vi "Timer Off Delay（SM).vi"(8 "error in":errorcluster caption="error IO", 10 "preset time (ms)":u32=1000, 11 "input":bool) -> (0 "error out":errorcluster caption="error IO", 2 "elapsed time (ms)":u32, 3 "output":bool)   [LabVIEW 2012, in "毫秒定时器.lvlib"]
uses:
  <vilib>/ptbypt/NI_PtbyPt.lvlib
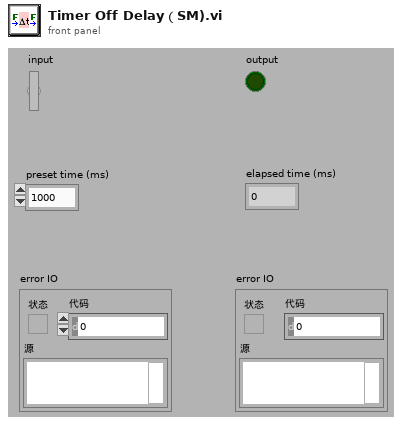
[diagram p1: front panel]
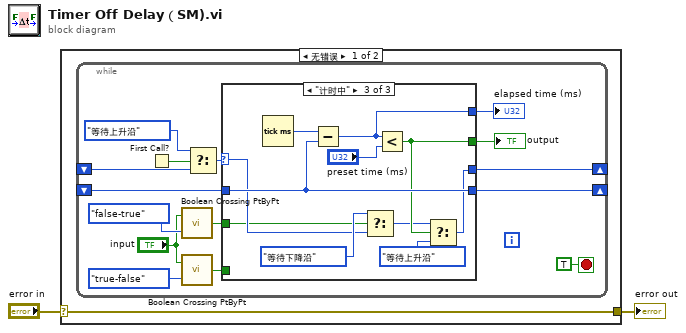
[diagram p0: block diagram]
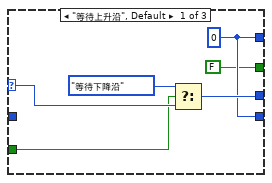
[diagram p2: hidden frame]
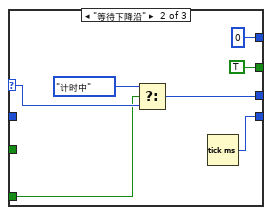
[diagram p3: hidden frame]
diagram:
  n1 = case shown="无错误" "error in" {
    selector: "error in" -> [w3 w43]
    tunnel: [w3 w43] -> w2
    frame No Error {
      n2 = while {
        shift-right: [w10] -> _
        shift-left: _ -> [w17]
        shift-right: [w11] -> _
        shift-left: _ -> [w13]
        stop <- TRUE stop-if-true
        n3 = First Call?() -> (First Call?: T/F=w16:bool)
        n4 = call <vilib>:"Boolean Crossing PtByPt.vi"("direction"=enum16{"either", "false-true", "true-false"}."false-true", "input"="input") -> ("crossing"=w5:bool)  [unwired: 1 in]
        n5 = call <vilib>:"Boolean Crossing PtByPt.vi"("direction"=enum16{"either", "false-true", "true-false"}."true-false", "input"="input") -> ("crossing"=w4:bool)  [unwired: 1 in]
        n6 = Select(t=enum16{"复位", "等待上升沿", "等待下降沿", "计时中"}."等待上升沿", s=w16, f=w17) -> (s? t:f=w14:enum16{"复位", "等待上升沿", "等待下降沿", "计时中"})
        n7 = case shown="\"计时中\"" w14 {
          selector: w14 -> [w24 w29 w37]
          tunnel: w13 -> [_ _ w39]
          tunnel: [FALSE ("input") TRUE ("input") w36] -> w12
          tunnel: [w21 u32 0 ("elapsed time (ms)") w40] -> w9
          tunnel: [w21 w30 w39] -> w11
          tunnel: [w22 w28 w34] -> w10
          tunnel: w5 -> [w20 _ w32]
          tunnel: w4 -> [_ w25 _]
          frame "等待上升沿", Default {
            w21 = u32 0 ("elapsed time (ms)")
            n8 = Select(t=enum16{"复位", "等待上升沿", "等待下降沿", "计时中"}."等待下降沿", s=w20, f=w24) -> (s? t:f=w22:enum16{"复位", "等待上升沿", "等待下降沿", "计时中"})
          }
          frame "等待下降沿" {
            n9 = Select(t=enum16{"复位", "等待上升沿", "等待下降沿", "计时中"}."计时中", s=w25, f=w29) -> (s? t:f=w28:enum16{"复位", "等待上升沿", "等待下降沿", "计时中"})
            n10 = Tick Count (ms)() -> (millisecond timer value=w30:u32)
          }
          frame "计时中" {
            n11 = Tick Count (ms)() -> (millisecond timer value=w42:u32)
            n12 = Subtract(x=w42, y=w39) -> (x-y=w40:u32)
            n13 = Select(t=enum16{"复位", "等待上升沿", "等待下降沿", "计时中"}."等待下降沿", s=w32, f=w37) -> (s? t:f=w35:enum16{"复位", "等待上升沿", "等待下降沿", "计时中"})
            n14 = Less?(x=w40, y="preset time (ms)") -> (x < y?=w36:bool)
            n15 = Select(t=w35, s=w36, f=enum16{"复位", "等待上升沿", "等待下降沿", "计时中"}."等待上升沿") -> (s? t:f=w34:enum16{"复位", "等待上升沿", "等待下降沿", "计时中"})
          }
        }
        "output" <- w12
        "elapsed time (ms)" <- w9
      }
    }
    frame Error {
    }
  }
  "error out" <- w2
